vi "Prev (SubVI).vi"(10 "Tab Control 2":T1(ring)) -> ()   [LabVIEW 2019]
uses:
  Global/Global_1.vi
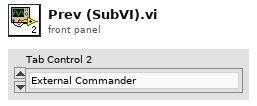
[diagram p1: front panel]
types:
  T1 = enum32{"External Commander", "Internal Commander", "Config Com", "Debug"}
  T2 = enum32{"External Commander", "Internal Commander", "Config Com", "Debug"}[]
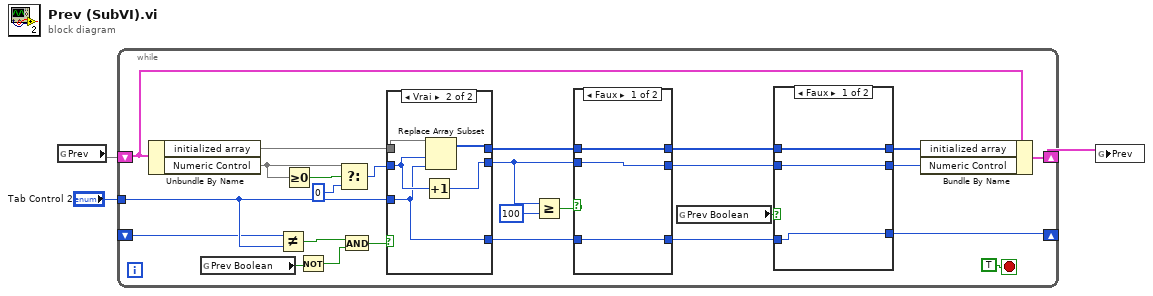
[diagram p0: block diagram]
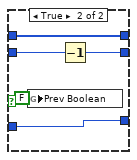
[diagram p2: hidden frame]
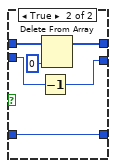
[diagram p3: hidden frame]
diagram:
  n1 = global read "Global_1.vi" "Prev"() -> (w2)
  n2 = while {
    tunnel: "Tab Control 2" -> [w27]
    shift-right: [w25] -> w1
    shift-left: w2 -> [w26]
    shift-right: [w15] -> _
    shift-left: _ -> [w12]
    stop <- TRUE stop-if-true
    n3 = Unbundle By Name(w26) -> ("initialized array"=w28, "Numeric Control"=w6)
    n4 = global read "Global_1.vi" "Prev Boolean"() -> (w11:bool)
    n5 = Not Equal?(x=w12, y=w27) -> (x != y?=w10:bool)
    n6 = Greater Or Equal To 0?(x=w6) -> (x >= 0?=w7:bool)
    n7 = Not(x=w11) -> (.not. x?=w9:bool)
    n8 = Select(t=w6, s=w7, f=0) -> (s? t:f=w4:i32)
    n9 = And(x=w10, y=w9) -> (x .and. y?=w8:bool)
    n10 = case shown="Vrai" w8 {
      tunnel: w28 -> [w49 w53]
      tunnel: w4 -> [w48 w51]
      tunnel: w27 -> [w47 w50]
      tunnel: [w49 w52] -> w22
      tunnel: [w48 w54] -> w21
      tunnel: [w47 w50] -> w13
      frame False {
      }
      frame True {
        n11 = Increment(x=w51) -> (x+1=w54:i32)
        n12 = Replace Array Subset(array=w53, new element=w50, index=w51) -> (w52:T2)
      }
    }
    n13 = Greater Or Equal?(x=w21, y=100) -> (x >= y?=w23:bool)
    n14 = case shown="Faux" w23 {
      tunnel: [w40 w45] -> w19
      tunnel: w22 -> [w40 w46]
      tunnel: [w39 w43] -> w18
      tunnel: w21 -> [w39 w44]
      tunnel: [w38 w41] -> w14
      tunnel: w13 -> [w38 w41]
      frame False {
      }
      frame True {
        n15 = Decrement(x=w44) -> (x-1=w43:i32)
        n16 = Delete From Array(array=w46, index=0) -> (array with subset deleted=w45:T2)  [unwired: 1 in, 1 out]
      }
    }
    n17 = global read "Global_1.vi" "Prev Boolean"() -> (w20:bool)
    n18 = case shown="Faux" w20 {
      tunnel: w19 -> [w32 w36]
      tunnel: w18 -> [w31 w35]
      tunnel: [w32 w36] -> w17
      tunnel: [w31 w34] -> w16
      tunnel: [w30 w33] -> w15
      tunnel: w14 -> [w30 w33]
      frame False {
      }
      frame True {
        n19 = global write "Global_1.vi" "Prev Boolean"(FALSE ("Prev Boolean")) -> ()
        n20 = Decrement(x=w35) -> (x-1=w34:i32)
      }
    }
    n21 = Bundle By Name(cluster=w26, "initialized array"=w17, "Numeric Control"=w16) -> (w25:cluster{})
  }
  n22 = global write "Global_1.vi" "Prev"(w1) -> ()
